vi "ztscopeM Check Status.vi"(4 "error in":errorcluster, 5 "name of VI":string, 6 "status (return code)":i32, 7 "instrument handle in":i32) -> (0 "error out":errorcluster, 3 "instrument handle out":i32)   [LabVIEW 2020, in "ZTScopeM.lvlib"]
doc: "Overview: \n\nThis VI converts error codes from LabWindows/CVI instrument drivers to standard LabVIEW error codes. If an error is detected the VI builds the appropriate error cluster that is readable by one of the error handlers supplied with LabVIEW. \n\nDetails:\n\n1. If an error has occurred in a previous VI, then the instrument handle and current error are passed through and nothing is executed.\n\n2. If no previous error has occurred, the status control is checked to see if an error occurred in the current subVI. Pass is 1 (no error) and 0 is fail (error).\n\n3. If no error has occurred in the current subVI, the instrument handle and current error are passed through and nothing is executed.\n\n4. If an error has occurred, the status is passed in the ZT4610 Errors subVI. This subVI returns an array of all of the errors that have occurred on the ZT4610 and the number that occurred.\n\n5. These error codes are passed to a For loop which iteratively retrieves the descriptions of each error and concatanates them into a single string.\n\n6. If more than one error has occurred, an additional string is concatanated into the final error description indication that \"multiple errors occurred\". \n\n7. The final error code is passed out to the error cluster along with a status of True and the error description string and this is fed to the error out."
uses:
  ZTScopeM.lvlib
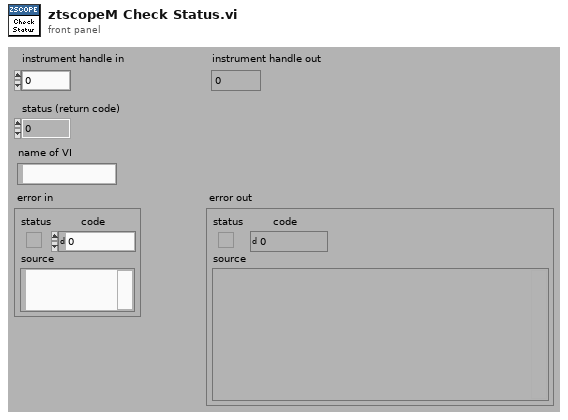
[diagram p1: front panel]
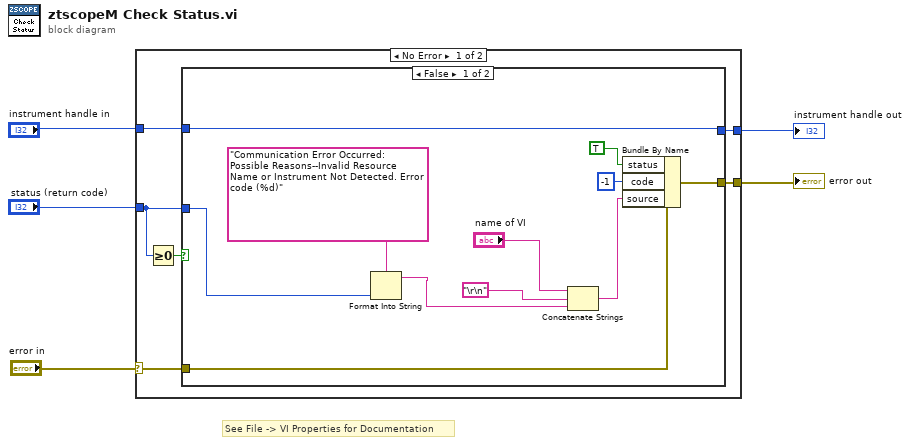
[diagram p0: block diagram]
diagram:
  # "See File -> VI Properties for Documentation"
  n1 = case shown="No Error" "error in" {
    selector: "error in" -> [w8 w26]
    tunnel: "status (return code)" -> [w11 _]
    tunnel: [w10 w26] -> w5
    tunnel: "instrument handle in" -> [w7 w25]
    tunnel: [w6 w25] -> w1
    frame No Error {
      n2 = Greater Or Equal To 0?(x=w11) -> (x >= 0?=w9:bool)
      n3 = case shown="False" w9 {
        tunnel: w8 -> [w18 w24]
        tunnel: [w22 w24] -> w10
        tunnel: w11 -> [w15 _]
        tunnel: w7 -> [w16 w23]
        tunnel: [w16 w23] -> w6
        frame False {
          n4 = Format Into String(format string="Communication Error Occurred: Possible Reasons--Invalid Resource Name or Instrument Not Detected. Error code (%d)", w15) -> (resulting string=w14:string)  [unwired: 2 in, 1 out]
          n5 = Concatenate Strings("name of VI", "\r\n", w14) -> (w20:string)
          n6 = Bundle By Name(cluster=w18, "status"=TRUE, "code"=-1, "source"=w20) -> (w22:errorcluster)
        }
        frame True {
        }
      }
    }
    frame Error {
    }
  }
  "error out" <- w5
  "instrument handle out" <- w1
